vi "Channel_Trim.vi"(0 "Piezo / nm":dbl[](array[numeric]), 1 "Femto in / V":dbl[](array[numeric]), 5 "Bias / V":dbl[](array[numeric]), 7 "G/G0":dbl[](array[numeric]), 9 "Error In":errorcluster, 11 "# Elements in queue":dbl, 12 "Aq Rt (20000) / Hz":dbl=20000.0 format="%0.2f") -> (3 "Femto out / V":dbl[](array[numeric]), 4 "Error Out":errorcluster, 6 "Piezo / nm Trim":dbl[](array[numeric]), 8 "Bias / V Trim":dbl[](array[numeric]), 10 "G/G0 Trim":dbl[](array[numeric]))   [LabVIEW 2025]
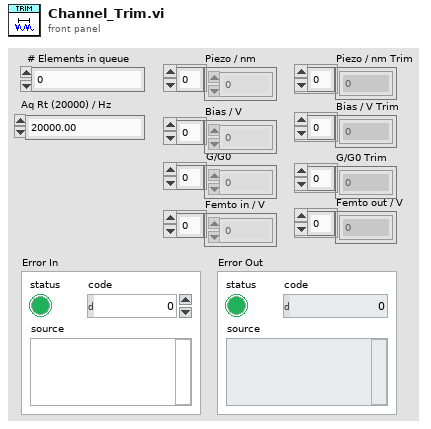
[diagram p1: front panel]
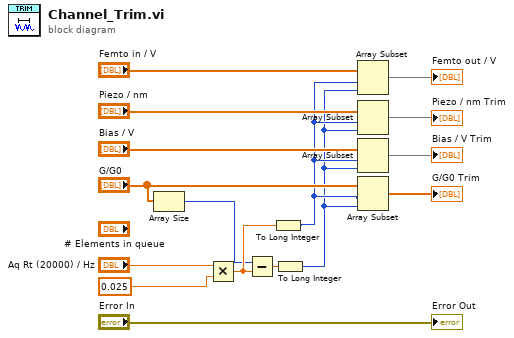
[diagram p0: block diagram]
diagram:
  n1 = Array Size(array="G/G0") -> (size(s)=w5:i32)
  n2 = Multiply(x="Aq Rt (20000) / Hz", y=0.025) -> (x*y=w7:dbl)
  n3 = Subtract(x=w5, y=w7) -> (x-y=w9:dbl)
  n4 = To Long Integer(number=w7) -> (32bit integer=w4:i32)
  n5 = To Long Integer(number=w9) -> (32bit integer=w3:i32)
  n6 = Array Subset(array="Femto in / V", index=w4, length=w3) -> (→"Femto out / V":dbl[])
  n7 = Array Subset(array="Piezo / nm", index=w4, length=w3) -> (→"Piezo / nm Trim":dbl[])
  n8 = Array Subset(array="Bias / V", index=w4, length=w3) -> (→"Bias / V Trim":dbl[])
  n9 = Array Subset(array="G/G0", index=w4, length=w3) -> (→"G/G0 Trim":dbl[])
  "Error Out" <- "Error In"
